vi "Get Timestamp.vi"(8 "error in (no error)":errorcluster, 9 "Data Type (default value)":timestamp, 10 "Offset":i32, 11 "JSON":string) -> (0 "error out":errorcluster, 1 "Timestamp":timestamp, 2 "Offset past match":i32)   [LabVIEW 2017, in "JSONtext.lvlib"]
uses:
  JSONtext.lvlib
  Parsing/Advance past String.vi
  String Subset.vi
  Strip Quotes and Unescape.vi
  Get Number Text.vi
  Parsing/NaN or null to Integer ERROR.vi
  Parsing/Advance past Number.vi
  Format Error.vi
  <vilib>/Utility/error.llb/Error Cluster From Error Code.vi
  Parsing/Parsing Error in converting to LabVIEW type.vi
  Unescape JSON string.vi
  <vilib>/JDP Science/JDP Science Common Utilities/Timestamp/JDP Timestamp.lvlib
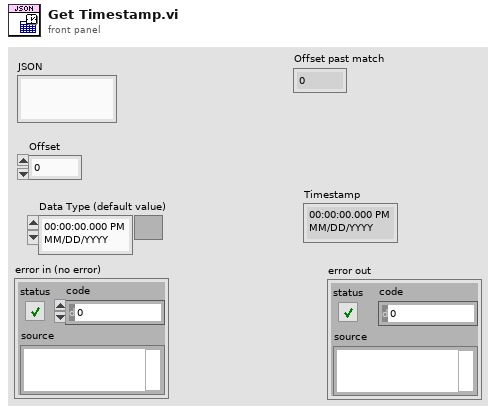
[diagram p1: front panel]
types:
  T1 = typedef "JSONtext.lvlib/Parsing State.ctl" = enum16{"Parser Error", "Object", "Array", "String", "Number/Other", "Leading Whitespace", "Object end", "Array end", "Value end"}
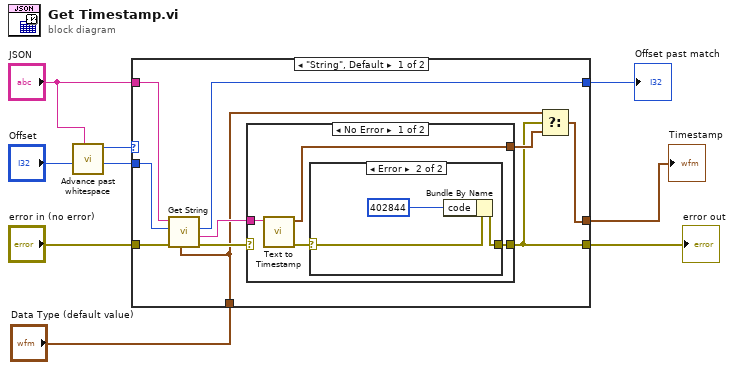
[diagram p0: block diagram]
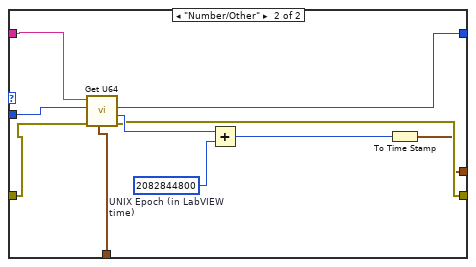
[diagram p4: hidden frame]
diagram:
  n1 = call "Advance past whitespace.vi"("JSON"="JSON", "Offset"="Offset") -> ("Offset of first non-whitespace"=w3:i32, "Parser State"=w2:T1)  [unwired: 8 in]
  n2 = case shown="\"String\", Default" w2 {
    tunnel: "error in (no error)" -> [w19 w33]
    tunnel: [w13 w31] -> w8
    tunnel: [w11 w32] -> w7
    tunnel: [w18 w30] -> w6
    tunnel: "JSON" -> [w17 w38]
    tunnel: w3 -> [w16 w37]
    tunnel: "Data Type (default value)" -> [w10 w29]
    frame "String", Default {
      n3 = call "Get String.vi"("LV Type"=w10, "error in (no error)"=w19, "Offset"=w16, "JSON"=w17) -> ("error out"=w12:errorcluster, "String"=w15:string, "Offset past match"=w18:i32)  [unwired: 5 in]
      n4 = case shown="No Error" w12 {
        selector: w12 -> [_ w28]
        tunnel: w15 -> [w23 _]
        tunnel: [w22 _] -> w14
        tunnel: [w20 w28] -> w11
        frame No Error {
          n5 = call <vilib>:"Text to Timestamp.vi"("Text Timestamp"=w23) -> ("error out"=w21:errorcluster, "Time Stamp"=w22:timestamp)  [unwired: 7 in, 2 out]
          n6 = case shown="Error" w21 {
            selector: w21 -> [w24 w27]
            tunnel: [w24 w26] -> w20
            frame No Error {
            }
            frame Error {
              n7 = Bundle By Name(cluster=w27, "code"=402844 ("error code (402840+)")) -> (w26:errorcluster)
            }
          }
        }
        frame Error {
        }
      }
      n8 = Select(t=w10, s=w11, f=w14) -> (s? t:f=w13:timestamp)
    }
    frame "Number/Other" {
      w36 = i64 2082844800  # UNIX Epoch (in LabVIEW time)
      n9 = call "Get U64.vi"("LV Type"=w29, "error in (no error)"=w33, "Offset"=w37, "JSON"=w38) -> ("error out"=w32:errorcluster, "Number"=w34:u64, "Offset past match"=w30:i32)  [unwired: 5 in]
      n10 = Add(x=w34, y=w36) -> (x+y=w35:u64)
      n11 = To Time Stamp(1:w35) -> (0:w31:timestamp)
    }
  }
  "error out" <- w7
  "Offset past match" <- w6
  "Timestamp" <- w8
